vi "is_valid_ref.vi"(11 "Value in":refnum<class "Value.lvclass">) -> (2 "valid-ref?":bool)   [LabVIEW 2020, in "toml_edit.lvlib" / "Value.lvclass"]
uses:
  Value.lvclass
  Value.lvclass/Value.ctl
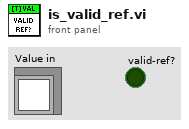
[diagram p1: front panel]
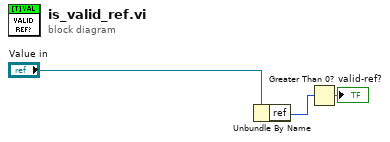
[diagram p0: block diagram]
diagram:
  n1 = Unbundle By Name("Value in") -> ("ref"=w2:u64)
  n2 = Greater Than 0?(x=w2) -> (x > 0?=→"valid-ref?":bool)
